vi "Gyro Acc Dec Back C1Stop.vi"(4 "Ref. light":sgl=12.0, 5 "Threshold to C1":i32=900, 6 "Ini. Degrees":sgl, 7 "Motor":cluster{"Port":T2, "Port":T2}={"Port"=1, "Port"=2} {"Port" items=["Port A", "Port B", "Port C", "Port D"]; "Port" items=["Port A", "Port B", "Port C", "Port D"]}, 8 "Threshold to De-acc":i32=700, 9 "De-acc":i32=10, 10 "Acc":i32=80, 11 "EV3 in":T1) -> (3 "EV3 out":T1)   [LabVIEW 2016]
uses:
  <vilib>/NXT/Block Support/NXT_OutputPort.ctl
  <vilib>/NXT/Subs/LVHSConnector.ctl
  <vilib>/NXT/LegoClasses/BrickReference/BrickReference.lvclass
  <vilib>/NXT/Block Support/NXT_InputPort.ctl
  <vilib>/NXT/NXTIO Xnodes/NXTIONodeSubVIs/LEGOResetMotors.vi
  <vilib>/NXT/Dual Mode Library/Motors/Rotation.vi
  <vilib>/NXT/Dual Mode Library/Sensors/EV3_Gyro_Angle.vi
  <vilib>/NXT/Dual Mode Library/Sensors/EV3_Color_Reflect.vi
  <vilib>/NXT/NXTIO Xnodes/NXTIONodeSubVIs/NXTMotorSteeringOn.vi
  <vilib>/NXT/NXTIO Xnodes/NXTIONodeSubVIs/NXTStopMotors.vi
  <vilib>/NXT/NXTIO Xnodes/NXTIOXNode/NXTIO.xnode
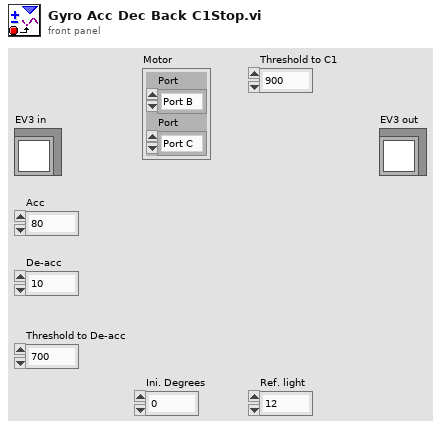
[diagram p1: front panel]
types:
  T1 = typedef "LVHSConnector.ctl" = refnum<class "BrickReference.lvclass">
  T2 = typedef "NXT_OutputPort.ctl" = u8
  T3 = typedef "NXT_InputPort.ctl" = u32
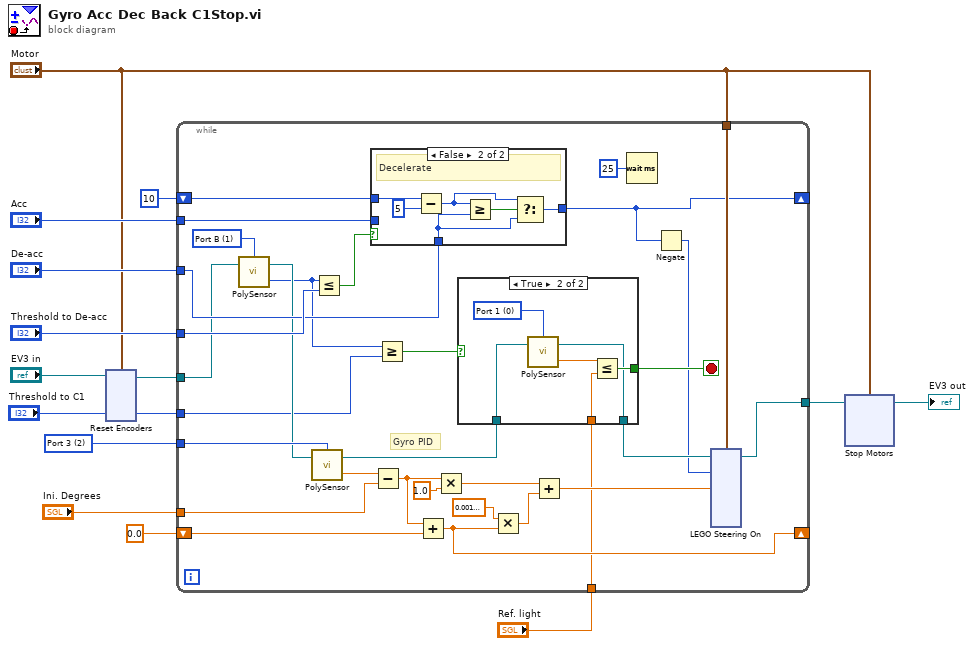
[diagram p0: block diagram]
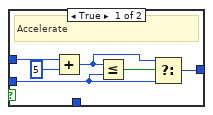
[diagram p3: hidden frame]
diagram:
  w12 = T3 2 items=["Port 1", "Port 2", "Port 3", "Port 4"] ("Port (Gyro)")
  n1 = xnode "Reset Encoders"("Motors"="Motor", "NXT/EV3"="EV3 in") -> ("NXT/EV3"=w9:T1)
  n2 = while {
    tunnel: w9 -> [w26]
    tunnel: w12 -> [w34]
    shift-right: [w42] -> _
    shift-left: sgl 0.0 -> [w43]
    tunnel: "Ini. Degrees" -> [w38]
    tunnel: [w33] -> w5
    tunnel: "Motor" -> [w36]
    shift-right: [w16] -> _
    shift-left: 10 -> [w30]
    tunnel: "De-acc" -> [w27]
    tunnel: "Acc" -> [w29]
    tunnel: "Threshold to De-acc" -> [w28]
    tunnel: "Threshold to C1" -> [w22]
    tunnel: "Ref. light" -> [w17]
    stop <- w20 stop-if-true
    w35 = T2 1 items=["Port A", "Port B", "Port C", "Port D"] ("Port (Port A)")
    # "Gyro PID"
    n3 = call-poly <vilib>:"PolySensor.vi"("NXT/EV3"=w26, "Port (Port A)"=w35) -> ("Angle of Rotation"=w23:i32, "NXT/EV3"=w25:T1)  [unwired: 1 in]
    n4 = call-poly <vilib>:"PolySensor.vi"("NXT/EV3"=w25, "Port (Port 1)"=w34) -> ("Degrees"=w45:sgl, "NXT/EV3"=w19:T1)  [unwired: 1 in]
    n5 = Less Or Equal?(x=w23, y=w28) -> (x <= y?=w24:bool)
    n6 = case shown="False" w24 {
      tunnel: w29 -> [w54 _]
      tunnel: w30 -> [w57 w63]
      tunnel: [w53 w60] -> w16
      tunnel: w27 -> [_ w59]
      frame True {
        # "Accelerate"
        n7 = Add(x=w57, y=5) -> (x+y=w55:i32)
        n8 = Less Or Equal?(x=w55, y=w54) -> (x <= y?=w56:bool)
        n9 = Select(t=w55, s=w56, f=w54) -> (s? t:f=w53:i32)
      }
      frame False {
        # "Decelerate"
        n10 = Subtract(x=w63, y=5) -> (x-y=w61:i32)
        n11 = Greater Or Equal?(x=w61, y=w59) -> (x >= y?=w62:bool)
        n12 = Select(t=w61, s=w62, f=w59) -> (s? t:f=w60:i32)
      }
    }
    n13 = Subtract(x=w45, y=w38) -> (x-y=w37:sgl)
    n14 = Greater Or Equal?(x=w23, y=w22) -> (x >= y?=w21:bool)
    n15 = Add(x=w37, y=w43) -> (x+y=w42:sgl)
    n16 = Multiply(x=w37, y=sgl 1.0 ("K_p")) -> (x*y=w40:sgl)
    n17 = case shown="True" w21 {
      tunnel: [_ w50] -> w20
      tunnel: w19 -> [w46 w49]
      tunnel: [w46 w48] -> w18
      tunnel: w17 -> [_ w47]
      frame False {
      }
      frame True {
        w52 = T3 0 items=["Port 1", "Port 2", "Port 3", "Port 4"] ("Port (Port 1)")
        n18 = call-poly <vilib>:"PolySensor.vi"("NXT/EV3"=w49, "Port (Port 1)"=w52) -> ("Scaled Value"=w51:sgl, "NXT/EV3"=w48:T1)  [unwired: 1 in]
        n19 = Less Or Equal?(x=w51, y=w47) -> (x <= y?=w50:bool)
      }
    }
    n20 = Multiply(x=sgl 0.001 ("K_i"), y=w42) -> (x*y=w39:sgl)
    n21 = Add(x=w40, y=w39) -> (x+y=w31:sgl)
    n22 = Wait (ms)(milliseconds to wait=u32 25) -> ()  [unwired: 1 out]
    n23 = Negate(x=w16) -> (-x=w15:i32)
    n24 = xnode "LEGO Steering On"("Steering 1"=w31, "Power 1"=w15, "Motors"=w36, "NXT/EV3"=w18) -> ("NXT/EV3"=w33:T1)
  }
  n25 = xnode "Stop Motors"("Motors"="Motor", "NXT/EV3"=w5) -> ("NXT/EV3"=→"EV3 out":T1)
